vi "Level 2 Tests.vi"(8 "error in (no error)":errorcluster, 10 "target alias":string="cRIO", 11 "configuration file path":path=path "/home/lvuser/RT_Exec_Timing.pcfg") -> (0 "error out":errorcluster, 1 "Results":T5(array[cluster]), 2 "Pass":bool, 3 "engine status":string)   [LabVIEW 2014]
uses:
  <vilib>/NI/Module Execution Interface/Engine Runtime/Execution States.ctl
  <vilib>/NI/Module Execution Interface/Engine Runtime/Fault.ctl
  <vilib>/NI/Tag Bus Module Framework/runtime/error classification.ctl
  CommonSubVIs/Framework/Flattened_Array/Get Parameter Value by Name I32.vi
  CommonSubVIs/Framework/Flattened_Array/Set Parameter Value by Name (I32).vi
  CommonSubVIs/Framework/Flattened_Array/Get Parameter Value by Name (U32).vi
  CommonSubVIs/Framework/Flattened_Array/Set Parameter Value by Name (U32).vi
  CommonSubVIs/Framework/Flattened_Array/Get Parameter Value by Name (Bool).vi
  CommonSubVIs/Framework/Flattened_Array/Set Parameter Value by Name (Bool).vi
  CommonSubVIs/Framework/Flattened_Array/Get Parameter Value by Name DBL.vi
  <vilib>/NI/Module Execution Interface/Engine Runtime/Engine Runtime Interface.lvclass
  <vilib>/NI/DCAF/Tag Editor Core/Framework Configuration Classes/target runtime/PL_Target Runtime.lvclass
  <vilib>/NI/Tag Bus Module Framework/runtime/TBM module execution interface.lvclass
panel:
  out "engine status cluster":T4(array[cluster])
  out "Done":bool
  out "Tab Control":enum32{"Jitter", "Additional Controls", "Other"}(tab)
  out "Loop Period (us)":u32=779
  out "Desired Repetitions":u32=100
  out "Warmup Iterations":i32=10
  out "Iterations":i32=1000
  out "CPU Cache":bool=TRUE
  out "Maximum Std Dev":dbl
  out "Maximum Jitter":dbl
  out "Flattened Array Out":string[](array[string])
  in  "Flattened Array in":string[](array[string])
  # "Settings"
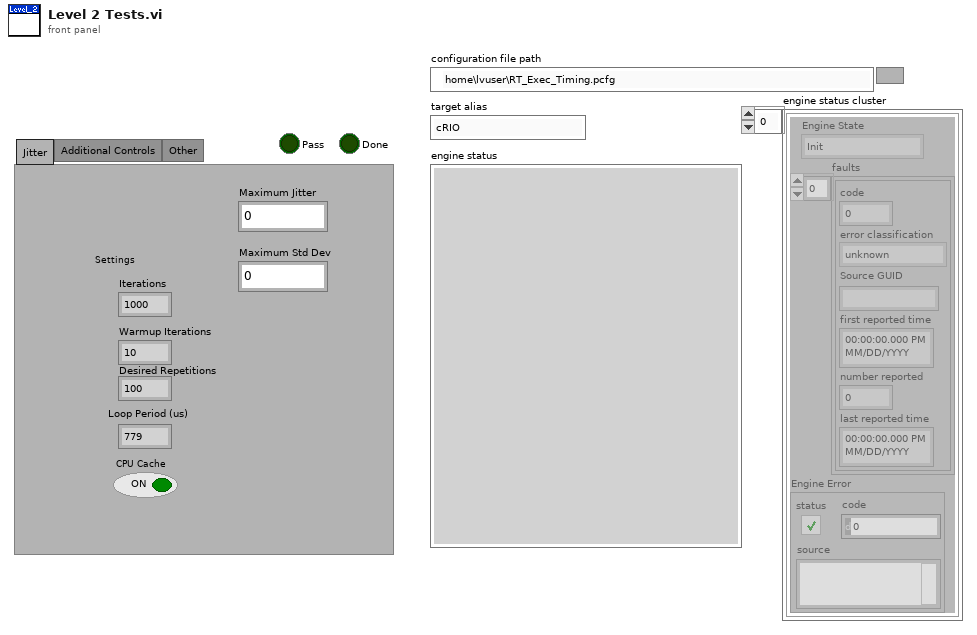
[diagram p1: front panel]
types:
  T1 = typedef "Engine Runtime Interface.lvclass/Execution States.ctl" = enum16{"Init", "Pre-Operational", "Safe-Operational", "Operational", "Stopped"}
  T2 = typedef "Engine Runtime Interface.lvclass/Fault.ctl" = cluster{"code":i32, "error classification":T3, "Source GUID":string, "first reported time":timestamp, "number reported":u32, "last reported time":timestamp}
  T3 = typedef "TBM module execution interface.lvclass/error classification.ctl" = enum16{"unknown", "none", "trivial", "recoverable", "critical"}
  T4 = cluster{"Engine State":T1, "faults":T2[], "Engine Error":errorcluster}[]
  T5 = cluster{"Name":string, "Value":dbl, "Units":string, "Format String":string}[]
  T6 = cluster{"Engine State":T1, "faults":T2[], "Engine Error":errorcluster}
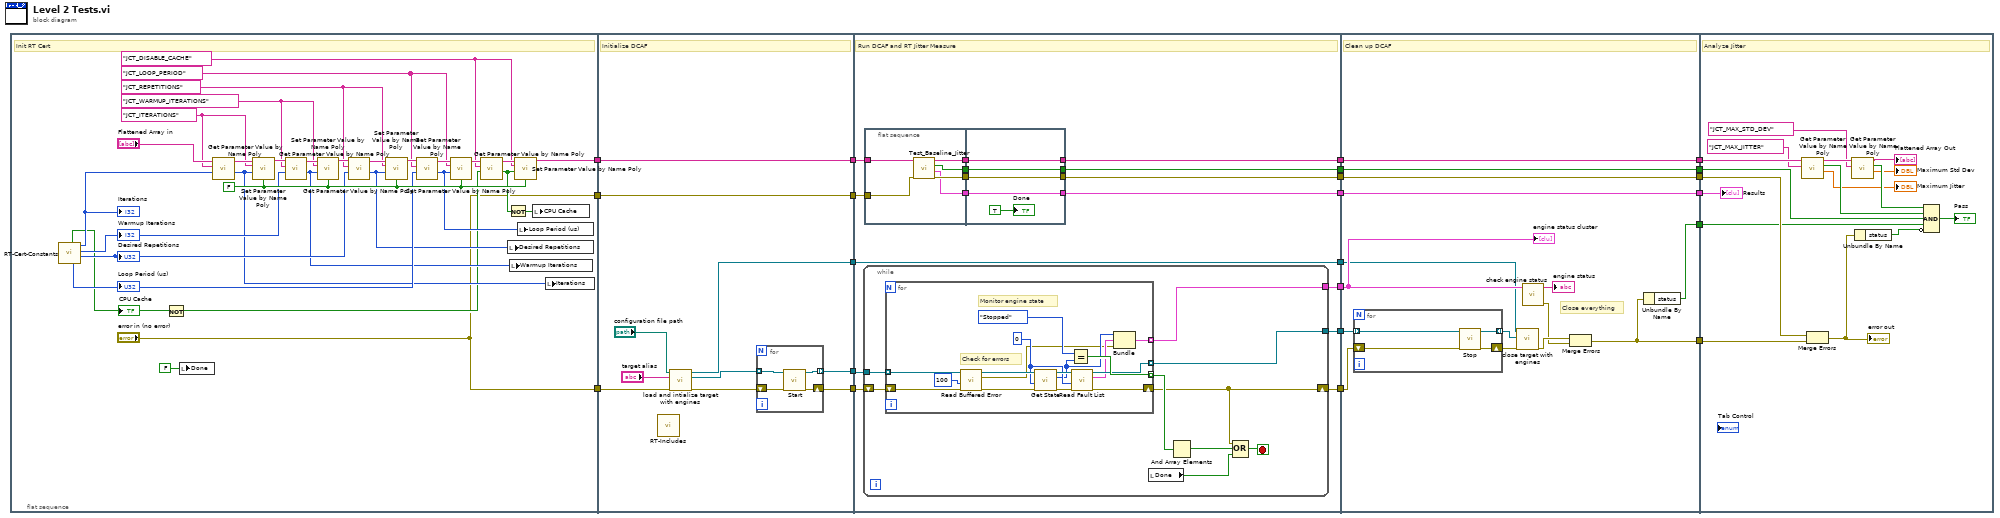
[diagram p0: block diagram]
diagram:
  n1 = flat-sequence "RTJC_L2_MAIN_FRAME" {
    tunnel: ["error in (no error)"] -> w16
    tunnel: [w41] -> w13
    tunnel: ["error in (no error)"] -> w9
    tunnel: w16 -> [w63]
    tunnel: [w63] -> w15
    tunnel: [w62] -> w14
    tunnel: w13 -> [w62]
    tunnel: w9 -> [w55]
    tunnel: [w57] -> w7
    tunnel: [w56] -> w4
    tunnel: [w54] -> w1
    tunnel: w15 -> [w83]
    tunnel: [w82] -> w21
    tunnel: [w81] -> w19
    tunnel: [w79] -> w18
    tunnel: w14 -> [w77]
    tunnel: [w76] -> w12
    tunnel: [w73] -> w8
    tunnel: w7 -> [w72]
    tunnel: [w70] -> w6
    tunnel: w4 -> [w69]
    tunnel: [w69] -> w3
    tunnel: [w68] -> w2
    tunnel: w1 -> [w71]
    tunnel: [w134] -> w22
    tunnel: w21 -> [w134]
    tunnel: [w133] -> w20
    tunnel: w19 -> [w133]
    tunnel: w18 -> [w132]
    tunnel: [w132] -> w17
    tunnel: w12 -> [w131]
    tunnel: [w131] -> w11
    tunnel: [w120] -> w10
    tunnel: w8 -> [w124]
    tunnel: w6 -> [w125]
    tunnel: [w121] -> w5
    tunnel: w3 -> [w123]
    tunnel: w2 -> [w122]
    tunnel: w22 -> [w155]
    tunnel: w20 -> [w154]
    tunnel: w17 -> [w147]
    tunnel: w11 -> [w153]
    tunnel: w10 -> [w142]
    tunnel: w5 -> [w141]
    frame #0 {
      w52 = FALSE
      w36 = "JCT_DISABLE_CACHE"
      w38 = "JCT_REPETITIONS"
      w39 = "JCT_WARMUP_ITERATIONS"
      w37 = "JCT_LOOP_PERIOD"
      w40 = "JCT_ITERATIONS"
      # "Init RT Cert"
      n2 = call "RT-Cert-Constants.vi"() -> ("Desired Repetitions"=w32:u32, "Warmup Iterations"=w29:i32, "Iterations"=w30:i32, "Loop Period (us)"=w34:u32, "CPU Cache"=w26:bool)  [unwired: 7 in]
      "Warmup Iterations" <- w29
      "Iterations" <- w30
      "Desired Repetitions" <- w32
      "Loop Period (us)" <- w34
      "CPU Cache" <- w26
      n3 = Not(x=w26) -> (.not. x?=w25:bool)
      n4 = local write "Done"(FALSE ("Done")) -> ()
      n5 = call-poly "Get Parameter Value by Name Poly.vi"("Default Value"=w30, "Parameter"=w40, "Parameter Array in"="Flattened Array in") -> ("Value"=w27:i32, "Parameter Array Out"=w43:string[])  [unwired: 5 in, 1 out]
      n6 = call-poly "Set Parameter Value by Name Poly.vi"("Parameter Array"=w43, "Parameter Name"=w40, "I32"=w27, "Override if found (T)"=w52) -> ("Parameter Array Out"=w50:string[])  [unwired: 8 in, 3 out]
      n7 = call-poly "Get Parameter Value by Name Poly.vi"("Default Value"=w29, "Parameter"=w39, "Parameter Array in"=w50) -> ("Value"=w28:i32, "Parameter Array Out"=w49:string[])  [unwired: 5 in, 1 out]
      n8 = call-poly "Set Parameter Value by Name Poly.vi"("Parameter Array"=w49, "Parameter Name"=w39, "I32"=w28, "Override if found (T)"=w52) -> ("Parameter Array Out"=w48:string[])  [unwired: 8 in, 3 out]
      n9 = call-poly "Get Parameter Value by Name Poly.vi"("Default Value"=w32, "Parameter"=w38, "Parameter Array in"=w48) -> ("Value"=w31:u32, "Parameter Array Out"=w47:string[])  [unwired: 5 in, 1 out]
      n10 = call-poly "Set Parameter Value by Name Poly.vi"("Parameter Array"=w47, "Parameter Name"=w38, "I32"=w31, "Override if found (T)"=w52) -> ("Parameter Array Out"=w46:string[])  [unwired: 8 in, 3 out]
      n11 = call-poly "Get Parameter Value by Name Poly.vi"("Default Value"=w34, "Parameter"=w37, "Parameter Array in"=w46) -> ("Value"=w33:u32, "Parameter Array Out"=w51:string[])  [unwired: 5 in, 1 out]
      n12 = call-poly "Set Parameter Value by Name Poly.vi"("Parameter Array"=w51, "Parameter Name"=w37, "I32"=w33, "Override if found (T)"=w52) -> ("Parameter Array Out"=w45:string[])  [unwired: 8 in, 3 out]
      n13 = call-poly "Get Parameter Value by Name Poly.vi"("Default Value"=w25, "Parameter"=w36, "Parameter Array in"=w45) -> ("Value"=w35:bool, "Parameter Array Out"=w44:string[])  [unwired: 5 in, 1 out]
      n14 = Not(x=w35) -> (.not. x?=w24:bool)
      n15 = local write "Desired Repetitions"(w31) -> ()
      n16 = local write "Warmup Iterations"(w28) -> ()
      n17 = call-poly "Set Parameter Value by Name Poly.vi"("Parameter Array"=w44, "Parameter Name"=w36, "Bool"=w35, "Override if found (T)"=w52) -> ("Parameter Array Out"=w41:string[])  [unwired: 8 in, 3 out]
      n18 = local write "Loop Period (us)"(w33) -> ()
      n19 = local write "CPU Cache"(w24) -> ()
      n20 = local write "Iterations"(w27) -> ()
    }
    frame #1 {
      # "Initialize DCAF"
      n21 = call "RT-Includes.vi"() -> ()  [unwired: 12 in]
      n22 = call <vilib>:"load and intialize target with engines.vi"("error in"=w55, "target alias"="target alias", "file path"="configuration file path") -> ("error out"=w61:errorcluster, "engine runtime interfaces"=w60:refnum<class "Engine Runtime Interface.lvclass">[], "target runtime"=w56:refnum<class "PL_Target Runtime.lvclass">)  [unwired: 6 in]
      n23 = for {
        tunnel: [w67] -> w57 mode=indexing
        tunnel: w60 -> [w64] mode=indexing
        shift-right: [w66] -> w54
        shift-left: w61 -> [w65]
        n24 = call-dynamic "Start.vi"("error in"=w65, "Engine Runtime Interface in"=w64) -> ("error out"=w66:errorcluster, "Engine Runtime Interface out"=w67:refnum<class "Engine Runtime Interface.lvclass">)  [unwired: 8 in]
      }
    }
    frame #2 {
      # "Run DCAF and RT Jitter Measure"
      n25 = while "RTJC_TS_LOOP" {
        tunnel: w72 -> [w90]
        shift-right: [w88] -> w73
        shift-left: w71 -> [w89]
        tunnel: [w87] -> w70
        tunnel: [w86] -> w68
        stop <- w84 stop-if-true
        n26 = for {
          tunnel: w90 -> [w108] mode=indexing
          tunnel: [w99] -> w86 mode=indexing
          tunnel: [w103] -> w92 mode=indexing
          shift-right: [w98] -> w88
          shift-left: w89 -> [w107]
          tunnel: [w93] -> w87 mode=indexing
          w97 = 0 ("timeout (-1)")
          # "Monitor engine state"
          # "Check for errors"
          n27 = call-dynamic "Read Buffered Error.vi"("error in"=w107, "timeout in ms (0)"=100, "Engine Runtime Interface in"=w108) -> ("error out"=w105:errorcluster, "Engine Error"=w94:errorcluster, "Engine Runtime Interface out"=w106:refnum<class "Engine Runtime Interface.lvclass">)  [unwired: 6 in]
          n28 = call-dynamic "Get State.vi"("error in"=w105, "timeout (-1)"=w97, "Engine Runtime Interface in"=w106) -> ("error out"=w101:errorcluster, "Engine State"=w96:T1, "Engine Runtime Interface out"=w100:refnum<class "Engine Runtime Interface.lvclass">)  [unwired: 6 in]
          n29 = Equal?(x=Execution_States."Stopped" ("Engine State"), y=w96) -> (x = y?=w103:bool)
          n30 = call-dynamic "Read Fault List.vi"("error in"=w101, "timeout (-1)"=w97, "Engine Runtime Interface in"=w100) -> ("error out"=w98:errorcluster, "faults"=w95:T2[], "Engine Runtime Interface out"=w99:refnum<class "Engine Runtime Interface.lvclass">)  [unwired: 6 in]
          n31 = Bundle("Engine State"=w96, "faults"=w95, "Engine Error"=w94) -> (w93:T6)  [unwired: 1 in]
        }
        n32 = local read "Done"() -> (w85:bool)
        n33 = And Array Elements(Boolean array=w92) -> (logical AND=w91:bool)
        n34 = Compound Arithmetic op=OR(w88, w91, w85) -> (w84:bool)
      }
      n35 = flat-sequence "RTJC_TS_FRAME" {
        tunnel: w83 -> [w113]
        tunnel: [w112] -> w80
        tunnel: [w110] -> w78
        tunnel: w77 -> [w114]
        tunnel: [w109] -> w75
        tunnel: [w111] -> w74
        tunnel: [w118] -> w82
        tunnel: w74 -> [w118]
        tunnel: [w117] -> w81
        tunnel: w80 -> [w117]
        tunnel: [w116] -> w79
        tunnel: w78 -> [w116]
        tunnel: [w115] -> w76
        tunnel: w75 -> [w115]
        frame #0 {
          n36 = call "Test_Baseline_Jitter.vi"("error in (no error)"=w113, "Falttened Array in"=w114) -> ("error out"=w112:errorcluster, "Results"=w111:T5, "Pass"=w110:bool, "Falttened Array Out"=w109:string[])  [unwired: 6 in]
        }
        frame #1 {
          "Done" <- TRUE
        }
      }
    }
    frame #3 {
      # "Close everything"
      # "Clean up DCAF"
      n37 = for {
        tunnel: w122 -> [w138] mode=indexing
        shift-right: [w135] -> w129
        shift-left: w124 -> [w137]
        tunnel: [w136] -> w130 mode=indexing
        n38 = call-dynamic "Stop.vi"("error in"=w137, "Engine Runtime Interface in"=w138) -> ("error out"=w135:errorcluster, "Engine Runtime Interface out"=w136:refnum<class "Engine Runtime Interface.lvclass">)  [unwired: 8 in]
      }
      n39 = call <vilib>:"close target with engines.vi"("error in"=w129, "Engine Runtime Interfaces"=w130, "Target Runtime"=w123) -> ("error out"=w127:errorcluster)  [unwired: 8 in]
      n40 = call "check engine status.vi"("engine status"=w125) -> ("error out"=w126:errorcluster, "JSON string"=→"engine status":string)  [unwired: 9 in]
      n41 = Merge Errors(w127, w126) -> (w121:errorcluster)
      n42 = Unbundle By Name(w121) -> ("status"=w120:bool)
      "engine status cluster" <- w125
    }
    frame #4 {
      # "Analyze Jitter"
      n43 = call-poly "Get Parameter Value by Name Poly.vi"("Parameter"="JCT_MAX_JITTER", "Parameter Array in"=w153) -> ("Value"=→"Maximum Jitter":dbl, "Found?"=w149:bool, "Parameter Array Out"=w151:string[])  [unwired: 6 in]
      n44 = Merge Errors(w154, w141) -> (w140:errorcluster)
      "error out" <- w140
      n45 = call-poly "Get Parameter Value by Name Poly.vi"("Parameter"="JCT_MAX_STD_DEV", "Parameter Array in"=w151) -> ("Value"=→"Maximum Std Dev":dbl, "Found?"=w148:bool, "Parameter Array Out"=→"Flattened Array Out":string[])  [unwired: 6 in]
      n46 = Unbundle By Name(w140) -> ("status"=w139:bool)
      n47 = Compound Arithmetic op=AND(w148, w149, w147, w142, invert w139) -> (→"Pass":bool)
      "Results" <- w155
    }
  }
